vi "Vision Research Phantom Series PhCon PhBlackReference.vi"(0 "CN in":u32=1, 5 "Error In (no error)":errorcluster, 7 "CallID":u32) -> (14 "CN out":u32=1, 19 "Error Out":errorcluster)   [LabVIEW 2013, in "VRI.lvlib"]
doc: "PhCon.dll\n\nPhBlackReference\nHRESULT PhBlackReference(UINT CN, PROGRESSCALLBACK pfnCallback);\n\nParameters Description\nCN (in) Camera number.\nCallID (in) Progress indicator.\nReturn HRESULT (0=Ok)\nComments You have to ask the operator to cover the lenses before\n calling this function. The software changes the acquisition\n parameters to the maximum resolution of this camera. If\n acceptable at this resolution, the frame rate and the\n exposure remain unchanged. AutoExposure and \n EDRExposure are disabled. PhCon acquires a number of\n raw images from the sensor in the darkness and averages\n them to find the pixel offsets. The new pixel offsets are \n stored in the stg file.\n The new black referende is usefull to compensate the\n change of the pixel offsets caused, for example, by a\n change in the sensor temperature. Better results can be\n obtained by calling PhBlackReferenceCI which does the \n calibration without changing the resolution or other\n acquisition parameters."
uses:
  VRI.lvlib
  Phantom DLLs/PhCon.dll
panel:
  # "For instructions on the use of this VI, press Ctrl+H to display the help window and move the mouse over the icon, controls, and indicators"
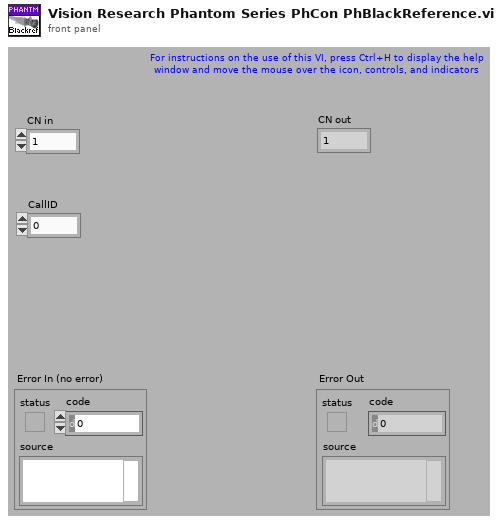
[diagram p1: front panel]
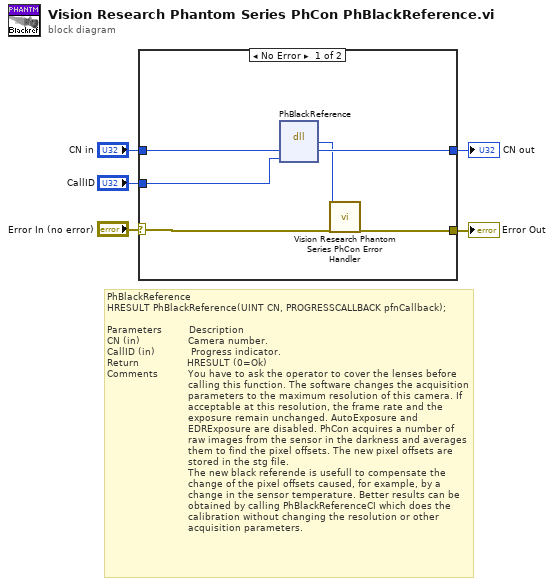
[diagram p0: block diagram]
diagram:
  # "PhBlackReference\nHRESULT PhBlackReference(UINT CN, PROGRESSCALLBACK pfnCallback);\n\nParameters         Description\nCN (in)                Camera number.\nCallID (in)            Progress indicator.\nReturn                HRESULT (0=Ok)\nComments          You have to ask the operator to cover the lenses before\n                           calling this function. The software changes the acquisition\n                           parameters to the maximum resolution of this camera. If\n                           acceptable at this resolution, the frame rate and the\n                           exposure remain unchanged. AutoExposure and  \n                           EDRExposure are disabled. PhCon acquires a number of\n                           raw images from the sensor in the darkness and averages\n                           them to find the pixel offsets. The new pixel offsets are \n                           stored in the stg file.\n                           The new black referende is usefull to compensate the\n                           change of the pixel offsets caused, for example, by a\n                           change in the sensor temperature. Better results can be\n                           obtained by calling PhBlackReferenceCI which does the \n                           calibration without changing the resolution or other\n                           acquisition parameters."
  n1 = case shown="No Error" "Error In (no error)" {
    selector: "Error In (no error)" -> [w11 w12]
    tunnel: [w10 w12] -> w4
    tunnel: "CN in" -> [w9 _]
    tunnel: [w8 _] -> w2
    tunnel: "CallID" -> [w7 _]
    frame No Error {
      n2 = dll-call lib="C:/Projects/SDK/32-bit/Vision Research Phantom Series Labview Driver/Phantom DLLs/PhCon.dll" fn="PhBlackReference"("CN"=w9, "CallID"=w7) -> ("HRESULT"=w6:i32, "CN"=w8:u32)  [unwired: 4 in, 2 out]
      n3 = call "Vision Research Phantom Series PhCon Error Handler.vi"("ErrNo"=w6, "Error In (no error)"=w11) -> ("Error Out"=w10:errorcluster)  [unwired: 17 out]
    }
    frame Error {
    }
  }
  "Error Out" <- w4
  "CN out" <- w2
